vi "get_is_data_named.vi"(11 "TypeDescriptor in":refnum<class "TypeDescriptor.lvclass">) -> (2 "is_named?":bool, 3 "TypeDescriptor out":refnum<class "TypeDescriptor.lvclass">)   [LabVIEW 2020, in "lvdata.lvlib" / "type_descriptor.lvlib" / "TypeDescriptor.lvclass"]
uses:
  TypeDescriptor.lvclass
  C:/projects/OpenG-Variant-Data-Library/source/library/Bytes/Bytes.lvclass
  Bytes/Bytes.lvclass/Bytes.ctl
  Bytes/from_byte_array.vi
  Bytes/Bytes.lvclass
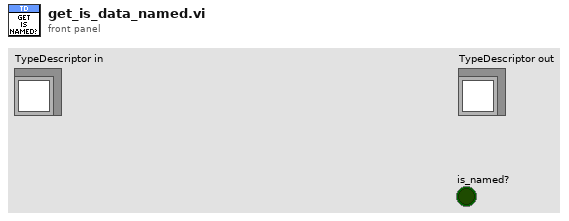
[diagram p1: front panel]
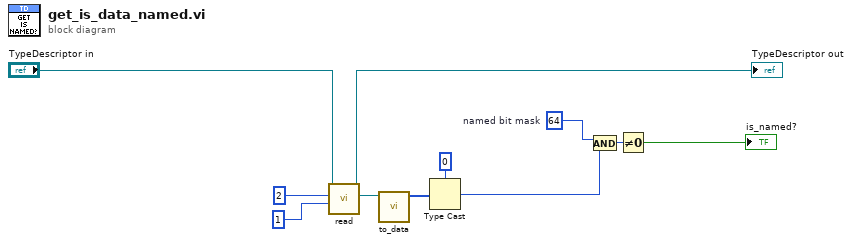
[diagram p0: block diagram]
diagram:
  w3 = u8 64  # named bit mask
  n1 = call "read.vi"("length (-1: rest)"=1, "offset (-1: current position)"=2, "Bytes in"="TypeDescriptor in") -> ("Bytes read"=w7:refnum<class "Bytes.lvclass">, "Bytes out"=→"TypeDescriptor out":refnum<class "TypeDescriptor.lvclass">)  [unwired: 7 in]
  n2 = call "to_data.vi"("Bytes in"=w7) -> ("byte array"=w6:u8[])  [unwired: 10 in]
  n3 = Type Cast(type=u8 0 ("u8"), x=w6) -> (*(type *) &x=w2:u8)
  n4 = And(x=w3, y=w2) -> (x .and. y?=w4:u8)
  n5 = Not Equal To 0?(x=w4) -> (x != 0?=→"is_named?":bool)
